vi "Maya2000 - Close all.vi"(8 "error in (no error)":errorcluster, 10 "Maya reference in":refnum<k24>) -> (0 "error out":errorcluster, 2 ".NET Refnum out":refnum<k24>)   [LabVIEW 2016]
uses:
  C:/Program Files/Ocean Optics/OmniDriver/OOI_HOME/NETOmniDriver-NET40.dll
  Program Files/Ocean Optics/OmniDriver/OOI_HOME/NETOmniDriver-NET40.dll
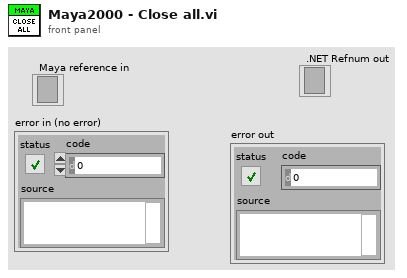
[diagram p1: front panel]
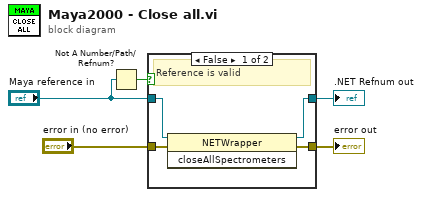
[diagram p0: block diagram]
diagram:
  n1 = Not A Number/Path/Refnum?(number/path/refnum="Maya reference in") -> (NaN/Path/Refnum?=w2:bool)
  n2 = case shown="False" w2 {
    tunnel: "error in (no error)" -> [w8 w10]
    tunnel: [w9 w11] -> w4
    tunnel: "Maya reference in" -> [w7 w11]
    tunnel: [w6 w10] -> w1
    frame False {
      # "Reference is valid"
      n3 = invoke class="NETWrapper" method="closeAllSpectrometers"(reference=w7, error in=w8) -> (reference out=w9:refnum<k24>, error out=w6:errorcluster)  [unwired: 1 in, 1 out]
    }
    frame True {
      # "Not a valid reference"
    }
  }
  ".NET Refnum out" <- w4
  "error out" <- w1
